vi "SHIFTER.vi"() -> (8 "SHIFTER DATA":T1 {"Display Data"."Wash Progress" scale=0.0..6.0})   [LabVIEW 2015, in "Car Wash.lvlib"]
uses:
  Car Wash.lvlib
  TypeDef - SHIFTER.ctl
  Dependencies.llb/Exit Event Ref.ctl
  Dependencies.llb/TLB`_Dependencies.lvlib
  State Declaration.ctl
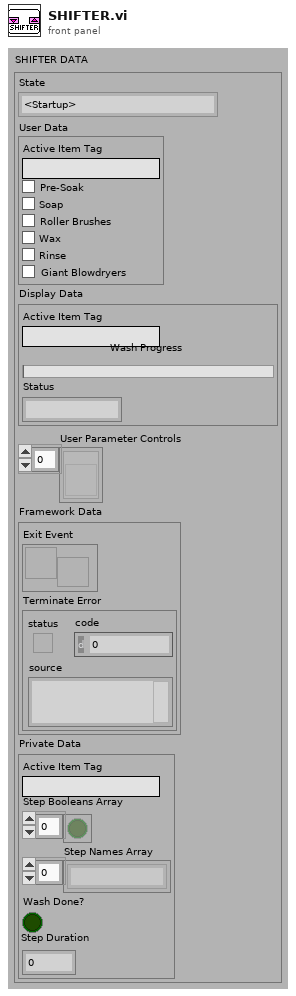
[diagram p1: front panel]
types:
  T1 = typedef "Car Wash.lvlib/TypeDef - SHIFTER.ctl" = cluster{"State":T2, "User Data":cluster{"Active Item Tag":string, "Pre-Soak":bool, "Soap":bool, "Roller Brushes":bool, "Wax":bool, "Rinse":bool, "Giant Blowdryers":bool}, "Display Data":cluster{"Active Item Tag":string, "Wash Progress":i32, "Status":string}, "User Parameter Controls":refnum<vi>[], "Framework Data":cluster{"Exit Event":T3, "Terminate Error":errorcluster}, "Private Data":cluster{"Active Item Tag":string, "Step Booleans Array":bool[], "Step Names Array":string[], "Wash Done?":bool, "Step Duration":i32}}
  T2 = typedef "Car Wash.lvlib/State Declaration.ctl" = enum16{"<Startup>", "Idle", "Washing", "<Shutdown>"}
  T3 = typedef "Car Wash.lvlib/TLB`_Dependencies.lvlib/Exit Event Ref.ctl" = refnum<user-event>
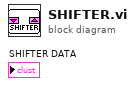
[diagram p0: block diagram]
diagram:
